vi "lab1 parte 2 ex 2.vi"() -> ()   [LabVIEW 2020]
uses:
  <vilib>/MakerHub/LINX/Public/Peripherals/Analog/Analog Read 1 Chan.vi
  <vilib>/MakerHub/LINX/Public/Peripherals/PWM/PWM Set Duty Cycle 1 Chan.vi
  <vilib>/MakerHub/LINX/Public/Peripherals/Analog/Analog Read N Chans.vi
  <vilib>/MakerHub/LINX/Private/Local IO/LinxAnalogRead.vi
  <vilib>/MakerHub/LINX/Public/Utilities/Check Channel.vi
  <vilib>/MakerHub/LINX/Public/Utilities/Open Serial.vi
  <vilib>/MakerHub/LINX/Private/Utilties/Generate Error.vi
  <vilib>/MakerHub/LINX/Public/Peripherals/PWM/PWM Set Duty Cycle N Chans.vi
  <vilib>/MakerHub/LINX/LMH-LINX.lvlib
panel:
  out "Error Out":errorcluster
  out "Thermometer":dbl(slide) scale=0.0..35.0
  out "Analog Input":dbl
  in  "stop":bool
  in  "Serial Port":refnum<visa-resource-name>
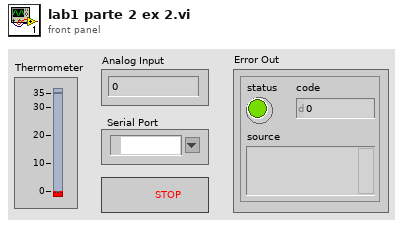
[diagram p1: front panel]
types:
  T1 = typedef "LMH-LINX.lvlib/LINX Ref.ctl" = cluster{"IO":T2, "Interface":T3, "LINX Device Config":T4}
  T2 = typedef "LMH-LINX.lvlib/Platform.ctl" = enum16{"Remote", "Local"}
  T3 = typedef "LMH-LINX.lvlib/Interface.ctl" = enum16{"Serial", "TCP"}
  T4 = typedef "LMH-LINX.lvlib/Device.lvlib/LINX Device Config.ctl" = cluster{"Interface":T3, "COM Port":refnum<visa-resource-name>, "TCP Configuration":T5, "Device Family":u8, "Device ID":u8, "Device Name":string, "TCP Ref":refnum<k5>, "Channels":T6}
  T5 = typedef "LMH-LINX.lvlib/Device.lvlib/TCP Config.ctl" = cluster{"IP Address":string, "Port":u16}
  T6 = typedef "LMH-LINX.lvlib/Channels.ctl" = cluster{"DI":u8[], "DO":u8[], "AI":u8[], "AO":u8[], "PWM":u8[], "QE":u8[], "UART":u8[], "I2C 2":u8[], "SPI":u8[], "CAN":u8[], "Servo":u8[], "AI Ref (V)":dbl, "AI Resolution (Bits)":u8, "AO Ref (V)":dbl, "AO Resolution (Bits)":u8}
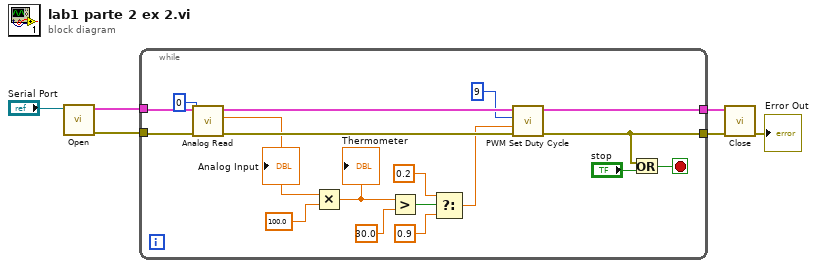
[diagram p0: block diagram]
diagram:
  n1 = call-poly <vilib>:"Open.vi"("Serial Port"="Serial Port") -> ("Error Out"=w4:errorcluster, "LINX Resource"=w5:T1)  [unwired: 8 in, 1 out]
  n2 = while {
    tunnel: w5 -> [w24]
    tunnel: w4 -> [w23]
    tunnel: [w18] -> w3
    tunnel: [w7] -> w2
    stop <- w9 stop-if-true
    n3 = call-poly <vilib>:"Analog Read.vi"("Error In"=w23, "Analog Channel"=u8 0, "LINX Resource"=w24) -> ("Error Out"=w20:errorcluster, "Voltage"=w17:dbl, "LINX Resource"=w21:T1)  [unwired: 5 in, 1 out]
    "Analog Input" <- w17
    n4 = Multiply(x=w17, y=100.0) -> (x*y=w15:dbl)
    "Thermometer" <- w15
    n5 = Greater?(x=w15, y=30.0) -> (0:w13:bool)
    n6 = Select(t=0.2, s=w13, f=0.9) -> (s? t:f=w10:dbl)
    n7 = call-poly <vilib>:"PWM Set Duty Cycle.vi"("Error In"=w20, "Duty Cycle (0-1)"=w10, "PWM Channel"=u8 9, "LINX Resource"=w21) -> ("Error Out"=w7:errorcluster, "LINX Resource"=w18:T1)  [unwired: 6 in]
    n8 = Or(x=w7, y="stop") -> (x .or. y?=w9:bool)
  }
  n9 = call <vilib>:"Close.vi"("Error In"=w2, "LINX Resource"=w3) -> ("Error Out"=→"Error Out":errorcluster)  [unwired: 9 in]
